vi "Excel Save Certification.vi"(4 "성적서 파일 경로":path, 5 "부록용":bool, 6 "성적서 파일명":string, 7 "시트잠금?":bool, 8 "에러 입력":errorcluster caption="에러 입력(에러 없음)", 9 "세부분류코드":string, 11 "test":string) -> (0 "에러 출력":errorcluster)   [LabVIEW 2020]
uses:
  <vilib>/Utility/NIReport.llb/NI_report.lvclass
  <vilib>/Utility/NIReport.llb/Report Type.ctl
  Controls/Cmd_File path.ctl
  Controls/Cmd_File Type.ctl
  <vilib>/Utility/error.llb/DialogType.ctl
  Variables/Global_Cal STD.vi
  Variables/Global_Cal Info.vi
  <vilib>/Utility/error.llb/Error Cluster From Error Code.vi
  <vilib>/addons/_office/excel.llb/Excel Get Data (str).vi
  <vilib>/ErrorRing/Error Ring.xnode
  <vilib>/Utility/NIReport.llb/Excel/NI_Excel.lvclass
  <vilib>/addons/_office/NI_ReportGenerationToolkit.lvlib
  <vilib>/Utility/NIReport.llb/NI_ReportGenerationCore.lvlib
panel:
  out "Comm":string
  out "Pass/Fail":string
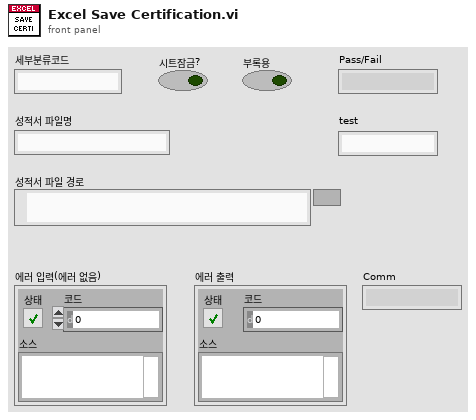
[diagram p1: front panel]
types:
  T1 = enum16{"Template Open", "File Save", "File Check", "End"}
  T2 = typedef "NI_ReportGenerationCore.lvlib/Report Type.ctl" = enum16{"HTML", "Word", "Excel"}
  T3 = enum16{"maximized", "minimized", "normal", "no change"}
  T4 = typedef "Cmd_File Type.ctl" = enum16{"엑셀", "엑셀(2003)", "텍스트", "설정", "2진", "VI", "CSV", "LOG", "폴더"}
  T5 = typedef "Cmd_File path.ctl" = enum16{"에러로그", "데이터파일경로", "성적서원본", "지난성적서", "Data Files", "경로생성", "Updater", "Template", "설정파일경로", "FTP Upload", "Update 경로", "어플리케이션"}
  T6 = typedef "Clst_Cal Info Global.ctl" = cluster{"등록번호":string, "의뢰기관":string, "기기명":string, "제작회사":string, "형식":string, "기기번호":string, "소분류코드":string, "세부분류코드":string, "교정주기":string, "접수번호":string, "교정일자":string, "교정절차서 1":string, "교정절차서 2":string, "교정절차서 3":string, "접수확인자":string, "인증교정자":string, "기술책임자":string, "KOLAS 유무":string, "진행상태":string, "의뢰기관코드":string, "입고형태":string, "영문성적서?":bool, "합불판정?":bool, "부록?":bool, "절차서번호 1":string, "절차서번호 2":string, "절차서번호 3":string, "교정방식":string, "부서명":string}
  T7 = typedef "DialogType.ctl" = u16
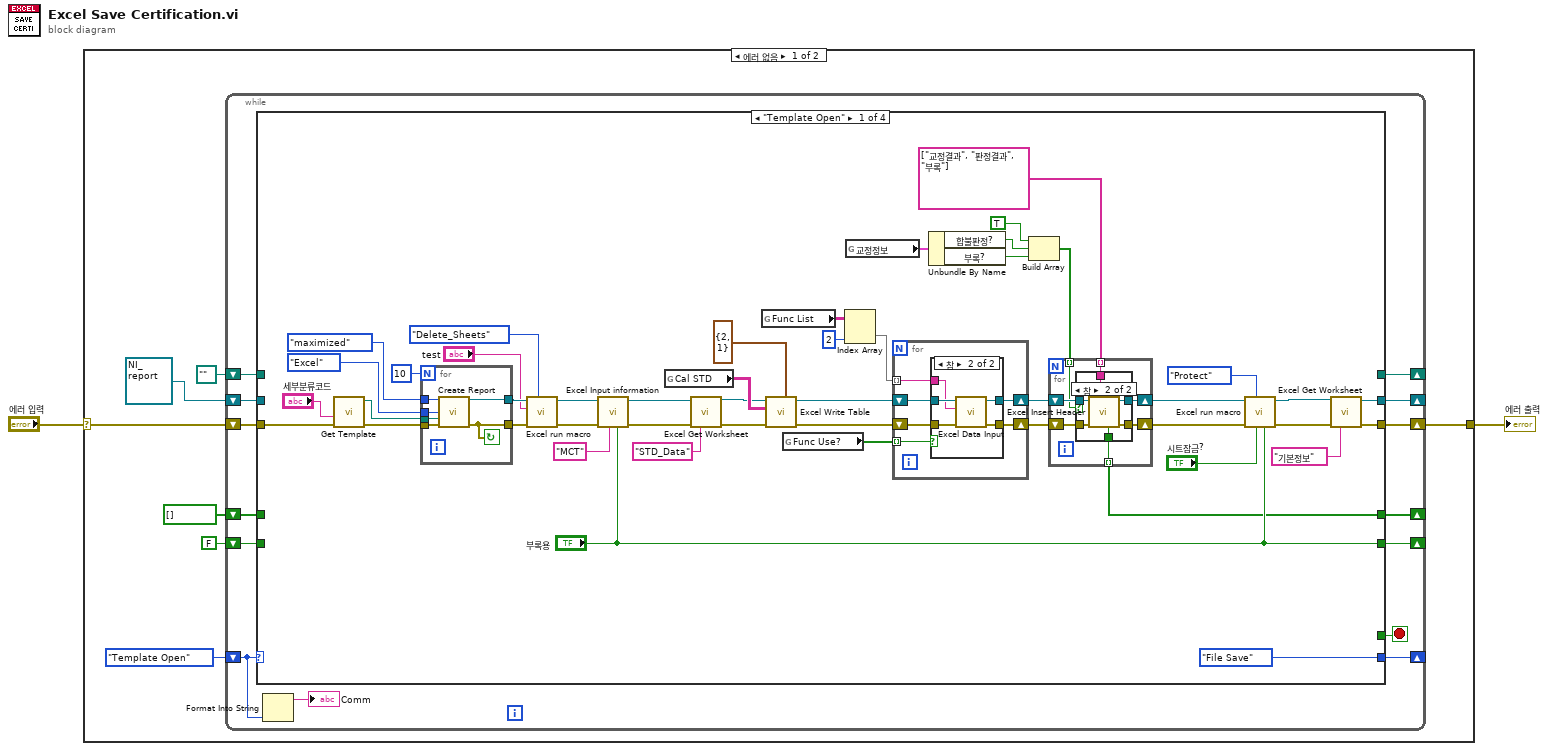
[diagram p0: block diagram]
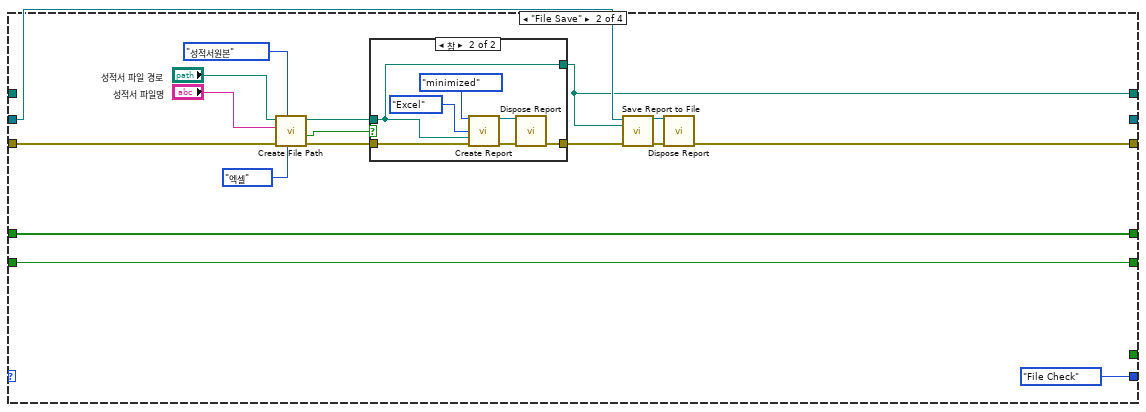
[diagram p4: hidden frame]
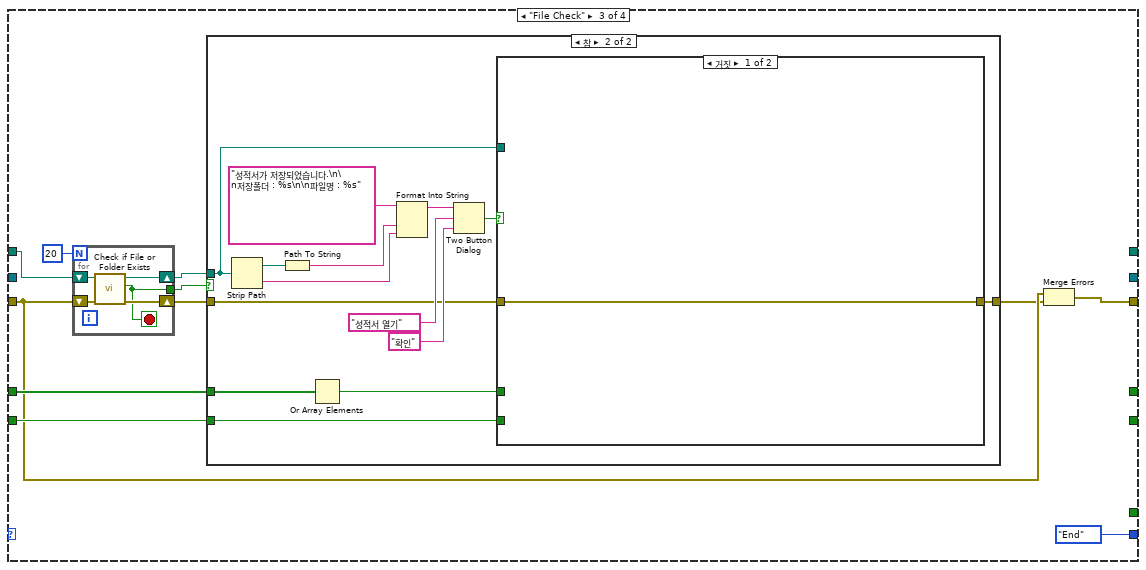
[diagram p6: hidden frame]
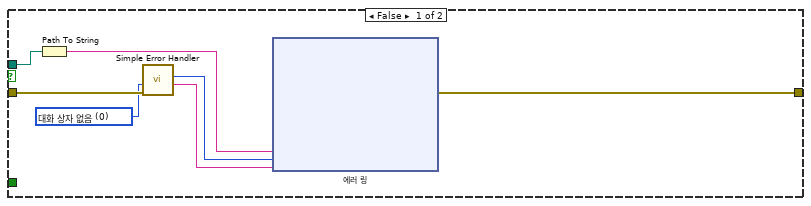
[diagram p7: hidden frame]
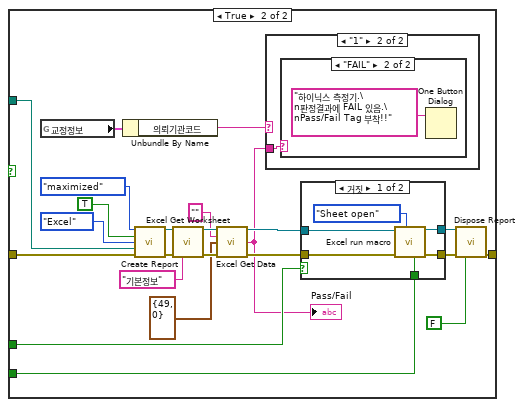
[diagram p8: hidden frame]
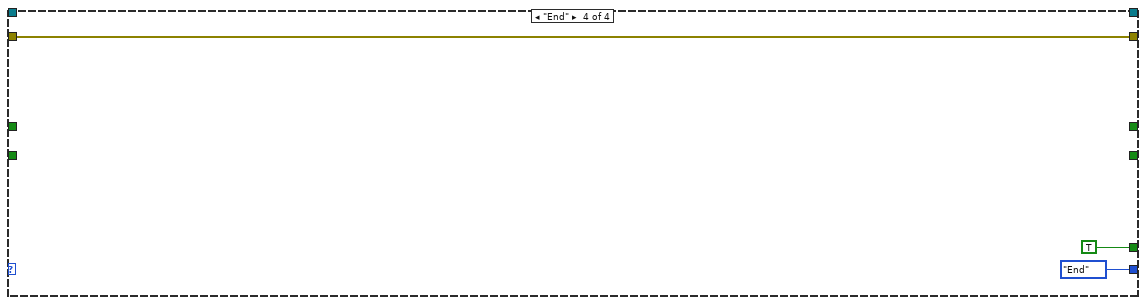
[diagram p12: hidden frame]
diagram:
  n1 = case shown="에러 없음" "에러 입력" {
    selector: "에러 입력" -> [w3 w214]
    tunnel: [w9 w214] -> w2
    frame No Error {
      n2 = while {
        shift-right: [w21] -> w9
        shift-left: w3 -> [w23]
        shift-right: [w22] -> _
        shift-left: refnum<class "NI_report.lvclass"> refnum ("report out") -> [w19]
        shift-right: [w20] -> _
        shift-left: T1."Template Open" -> [w11]
        shift-right: [w18] -> _
        shift-left: FALSE ("부록용") -> [w13]
        shift-right: [w17] -> _
        shift-left: path "" ("파일경로") -> [w16]
        shift-right: [w15] -> _
        shift-left: bool[] [] -> [w14]
        stop <- w12 stop-if-true
        n3 = case shown="\"Template Open\"" w11 {
          tunnel: w23 -> [w62 w120 w133 w213]
          tunnel: [w29 _ _ _] -> w22
          tunnel: [w28 w108 w134 w213] -> w21
          tunnel: [T1."File Save" T1."File Check" T1."End" T1."End"] -> w20
          tunnel: w19 -> [_ w110 _ _]
          tunnel: ["부록용" w106 _ _] -> w18
          tunnel: [_ w109 _ _] -> w17
          tunnel: w16 -> [_ _ w140 _]
          tunnel: [w25 w107 _ _] -> w15
          tunnel: w14 -> [_ w107 w136 _]
          tunnel: w13 -> [_ w106 w135 _]
          tunnel: [_ _ _ TRUE] -> w12
          frame "Template Open" {
            n4 = call "Get Template.vi"("에러 입력"=w62, "세부분류코드"="세부분류코드") -> ("에러 출력"=w69:errorcluster, "Templates Path"=w68:path)  [unwired: 8 in]
            n5 = for {
              N: 10 -> [_]
              tunnel: w69 -> [w104]
              tunnel: w68 -> [w103]
              tunnel: T3."maximized" ("window state (normal)") -> [w102]
              tunnel: Report_Type."Excel" ("report type") -> [w101]
              tunnel: [w100] -> w65
              tunnel: [w99] -> w66
              stop <- w100 continue-if-true
              n6 = call <vilib>:"Create Report.vi"("window state (normal)"=w102, "report type"=w101, "template (empty)"=w103, "error in (no error)"=w104) -> ("report out"=w99:refnum<class "NI_report.lvclass">, "error out"=w100:errorcluster)  [unwired: 10 in]
            }
            n7 = call "Excel run macro.vi"("Comm"=enum16{"Protect", "Delete_Sheets"}."Delete_Sheets", "error in"=w65, "test"="test", "report in"=w66) -> ("error out"=w59:errorcluster, "report out"=w58:refnum<class "NI_report.lvclass">)  [unwired: 6 in]
            n8 = call "Excel Input information.vi"("부록용"="부록용", "문자열"="MCT", "error in"=w59, "report in"=w58) -> ("error out"=w56:errorcluster, "report out"=w55:refnum<class "NI_report.lvclass">)  [unwired: 6 in]
            n9 = global read "Global_Cal STD.vi" "Cal STD"() -> (w52:string[][])
            n10 = call <vilib>:"Excel Get Worksheet.vi"("report in"=w55, "error in (no error)"=w56, "name (\"\")"="STD_Data" ("name (\"\")")) -> ("report out"=w51:refnum<class "NI_report.lvclass">, "error out"=w53:errorcluster)  [unwired: 11 in]
            n11 = global read "Global_Cal Info.vi" "Func List"() -> (w46:string[][])
            n12 = call "Excel Write Table.vi"("Address"=cluster{"Row":i32, "Column":i32} {"Row"=2, "Column"=1}, "error in"=w53, "table"=w52, "report in"=w51) -> ("error out"=w48:errorcluster, "report out"=w49:refnum<class "NI_report.lvclass">)  [unwired: 4 in, 2 out]
            n13 = global read "Global_Cal Info.vi" "Func Use?"() -> (w44:bool[])
            n14 = Index Array(array=w46, index (col)=2 ("비활성화된 인덱스 (열)")) -> (element=w45:string[])  [unwired: 1 in]
            n15 = global read "Global_Cal Info.vi" "교정정보"() -> (w39:T6)
            n16 = for {
              tunnel: w45 -> [w89] mode=indexing
              shift-right: [w88] -> w42
              shift-left: w48 -> [w91]
              shift-right: [w87] -> w43
              shift-left: w49 -> [w90]
              tunnel: w44 -> [w86] mode=indexing
              n17 = case shown="참" w86 {
                tunnel: w91 -> [w92 w98]
                tunnel: w90 -> [w93 w97]
                tunnel: w89 -> [_ w96]
                tunnel: [w92 w95] -> w88
                tunnel: [w93 w94] -> w87
                frame False {
                }
                frame True {
                  n18 = call "Excel Data Input.vi"("에러 입력"=w98, "Name"=w96, "NI_report 입력"=w97) -> ("에러 출력"=w95:errorcluster, "NI_report 출력"=w94:refnum<class "NI_report.lvclass">)  [unwired: 7 in]
                }
              }
            }
            n19 = Unbundle By Name(w39) -> ("합불판정?"=w41:bool, "부록?"=w38:bool)
            n20 = Build Array(TRUE ("원소"), w41, w38) -> (w37:bool[])
            n21 = for {
              tunnel: string[] ["교정결과", "판정결과", "부록"] -> [w73] mode=indexing
              shift-right: [w75] -> w36
              shift-left: w43 -> [w77]
              shift-right: [w74] -> w34
              shift-left: w42 -> [w76]
              tunnel: w37 -> [w72] mode=indexing
              tunnel: [w71] -> w25 mode=indexing
              n22 = case shown="참" w72 {
                tunnel: w77 -> [w79 w85]
                tunnel: w76 -> [w78 w84]
                tunnel: [w79 w83] -> w75
                tunnel: [w78 w82] -> w74
                tunnel: w73 -> [_ w81]
                tunnel: [_ w80] -> w71
                frame False {
                }
                frame True {
                  n23 = call "Excel Insert Header.vi"("시트명"=w81, "error in"=w84, "report in"=w85) -> ("error out"=w82:errorcluster, "report out"=w83:refnum<class "NI_report.lvclass">, "삭제에러"=w80:bool)  [unwired: 6 in]
                }
              }
            }
            n24 = call "Excel run macro.vi"("부록용"="부록용", "시트잠금?"="시트잠금?", "Comm"=enum16{"Protect", "Delete_Sheets"}."Protect", "error in"=w34, "report in"=w36) -> ("error out"=w31:errorcluster, "report out"=w30:refnum<class "NI_report.lvclass">)  [unwired: 5 in]
            n25 = call <vilib>:"Excel Get Worksheet.vi"("report in"=w30, "error in (no error)"=w31, "name (\"\")"="기본정보" ("name (\"\")")) -> ("report out"=w29:refnum<class "NI_report.lvclass">, "error out"=w28:errorcluster)  [unwired: 11 in]
          }
          frame "File Save" {
            n26 = call "Create File Path.vi"("파일타입"=Cmd_File_Type."엑셀", "항목"=Cmd_File_path."성적서원본", "에러 입력"=w120, "문자열 in"="성적서 파일명", "폴더명 in"="성적서 파일 경로") -> ("error out"=w116:errorcluster, "파일존재?"=w115:bool, "파일경로"=w114:path)  [unwired: 3 in, 1 out]
            n27 = case shown="참" w115 {
              tunnel: w116 -> [w123 w130]
              tunnel: [w123 w126] -> w111
              tunnel: w114 -> [w122 w125]
              tunnel: [w122 w125] -> w109
              frame False {
              }
              frame True {
                n28 = call <vilib>:"Create Report.vi"("window state (normal)"=T3."minimized", "report type"=Report_Type."Excel", "template (empty)"=w125, "error in (no error)"=w130) -> ("report out"=w127:refnum<class "NI_report.lvclass">, "error out"=w129:errorcluster)  [unwired: 10 in]
                n29 = call-dynamic "Dispose Report.vi"("report in"=w127, "error in (no error)"=w129) -> ("error out"=w126:errorcluster)  [unwired: 13 in]
              }
            }
            n30 = call-dynamic "Save Report to File.vi"("report in"=w110, "report file path"=w109, "error in (no error)"=w111) -> ("report out"=w112:refnum<class "NI_report.lvclass">, "error out"=w113:errorcluster)  [unwired: 11 in]
            n31 = call-dynamic "Dispose Report.vi"("report in"=w112, "error in (no error)"=w113) -> ("error out"=w108:errorcluster)  [unwired: 13 in]
          }
          frame "File Check" {
            n32 = for {
              N: 20 -> [_]
              shift-right: [w143] -> w139
              shift-left: w140 -> [w145]
              tunnel: [w142] -> w137
              shift-right: [w144] -> w138
              shift-left: w133 -> [w146]
              stop <- w142 stop-if-true
              n33 = call <vilib>:"Check if File or Folder Exists.vi"("error in (no error)"=w146, "path"=w145) -> ("error out"=w144:errorcluster, "file or folder exists?"=w142:bool, "dup path"=w143:path)  [unwired: 7 in]
            }
            n34 = case shown="참" w137 {
              tunnel: w139 -> [w148 w172]
              tunnel: w138 -> [w153 w171]
              tunnel: [w151 w170] -> w132
              tunnel: w136 -> [_ w165]
              tunnel: w135 -> [_ w163]
              frame False {
                w152 = T7 0 items=["대화 상자 없음", "확인 메시지", "메시지 지속 또는 정지", "확인 메시지 + 경고", "지속/정지 + 경고"] ("type of dialog (OK msg:1)")
                n35 = Path To String(path=w148) -> (string=w147:string)
                n36 = call <vilib>:"Simple Error Handler.vi"("type of dialog (OK msg:1)"=w152, "error in (no error)"=w153) -> ("code out"=w149:i32, "source out"=w150:string)  [unwired: 3 in, 3 out]
                n37 = xnode "에러 링"("파라미터 0"=w147, "파라미터 1"=w149, "파라미터 2"=w150) -> ("에러 출력"=w151:errorcluster)
              }
              frame True {
                n38 = Strip Path(path=w172) -> (stripped path=w176:path, name=w167:string)
                n39 = Path To String(path=w176) -> (string=w168:string)
                n40 = Or Array Elements(Boolean array=w165) -> (logical OR=w164:bool)
                n41 = Format Into String(format string="성적서가 저장되었습니다.\n\n저장폴더 : %s\n\n파일명 : %s" ("메시지"), w168, w167) -> (resulting string=w166:string)  [unwired: 2 in, 1 out]
                n42 = Two Button Dialog(message=w166, 1:"확인" ("거짓 버튼 이름(\"취소\")"), 2:"성적서 열기" ("참 버튼 이름(\"확인\")")) -> (T button?=w173:bool)
                n43 = case shown="거짓" w173 {
                  tunnel: w172 -> [_ w200]
                  tunnel: w171 -> [w177 w199]
                  tunnel: [w177 w196] -> w170
                  tunnel: w164 -> [_ w181]
                  tunnel: w163 -> [_ w180]
                  frame False {
                  }
                  frame True {
                    n44 = global read "Global_Cal Info.vi" "교정정보"() -> (w189:T6)
                    n45 = Unbundle By Name(w189) -> ("의뢰기관코드"=w188:string)
                    n46 = call <vilib>:"Create Report.vi"("window state (normal)"=T3."maximized", "display alerts? (F)"=TRUE, "report type"=Report_Type."Excel", "template (empty)"=w200, "error in (no error)"=w199) -> ("report out"=w187:refnum<class "NI_report.lvclass">, "error out"=w186:errorcluster)  [unwired: 9 in]
                    n47 = call <vilib>:"Excel Get Worksheet.vi"("report in"=w187, "error in (no error)"=w186, "name (\"\")"="기본정보" ("name (\"\")")) -> ("report out"=w193:refnum<class "NI_report.lvclass">, "error out"=w194:errorcluster)  [unwired: 11 in]
                    n48 = call-poly <vilib>:"Excel Get Data.vi"("report in"=w193, "data type"="", "start (0, 0)"=cluster{"start row":i32, "start column":i32} {"start row"=49, "start column"=0}, "error in (no error)"=w194) -> ("report out"=w185:refnum<class "NI_report.lvclass">, "data"=w178:string, "error out"=w184:errorcluster)  [unwired: 9 in]
                    "Pass/Fail" <- w178
                    n49 = case shown="\"1\"" w188 {
                      tunnel: w178 -> [_ w209]
                      frame Default {
                      }
                      frame "1" {
                        n50 = case shown="\"FAIL\"" w209 {
                          frame "거짓", Default {
                          }
                          frame "FAIL" {
                            n51 = One Button Dialog(message="하이닉스 측정기.\n판정결과에 FAIL 있음.\nPass/Fail Tag 부착!!" ("메시지")) -> ()  [unwired: 1 in, 1 out]
                          }
                        }
                      }
                    }
                    n52 = case shown="거짓" w181 {
                      tunnel: w185 -> [w206 w208]
                      tunnel: w184 -> [w205 w207]
                      tunnel: [w204 w208] -> w183
                      tunnel: [w203 w207] -> w182
                      tunnel: w180 -> [w201 _]
                      frame False {
                        n53 = call "Excel run macro.vi"("부록용"=w201, "Comm"=enum16{"Protect", "Delete_Sheets", "Sheet open"}."Sheet open", "error in"=w205, "report in"=w206) -> ("error out"=w203:errorcluster, "report out"=w204:refnum<class "NI_report.lvclass">)  [unwired: 6 in]
                      }
                      frame True {
                      }
                    }
                    n54 = call-dynamic "Dispose Report.vi"("report in"=w183, "error in (no error)"=w182, "close report? (T)"=FALSE) -> ("error out"=w196:errorcluster)  [unwired: 12 in]
                  }
                }
              }
            }
            n55 = Merge Errors(w133, w132) -> (w134:errorcluster)
          }
          frame "End" {
          }
        }
        n56 = Format Into String(w11) -> (resulting string=→"Comm":string)  [unwired: 3 in, 1 out]
      }
    }
    frame Error {
    }
  }
  "에러 출력" <- w2
